vi "MAIN_TL_wait_cycle_end.vi"(6 "Gauge Refnum":refnum<vi>, 7 "# repetition":i32, 8 "error in":errorcluster, 9 "variant":variant, 10 "t0":dbl, 11 "# cycle":i32) -> (0 "error out":errorcluster, 1 "task":T1, 4 "# cycles":i32, 5 "To":dbl)   [LabVIEW 2015]
uses:
  CONTROLS/Q_main_element.ctl
  GLOBAL/Global_ABORT.vi
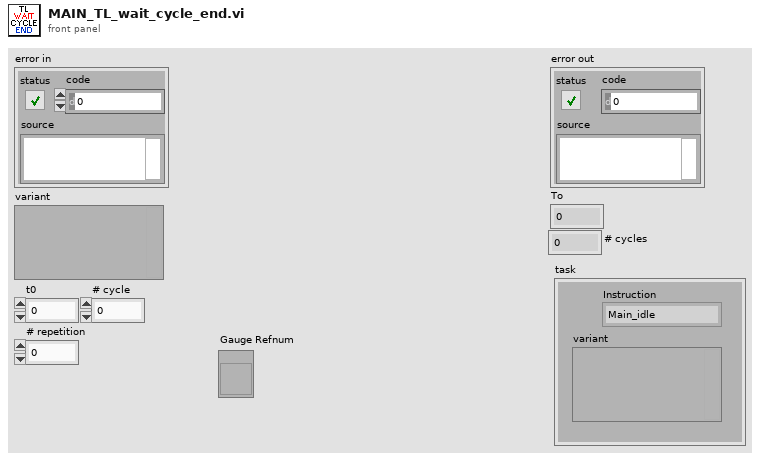
[diagram p1: front panel]
types:
  T1 = typedef "Q_main_element.ctl" = cluster{"variant":variant, "Instruction":enum16{"Main_idle", "Main_initialize", "Main_initialize_TDMS", "Main_initialize_Queue", "Main_error", "Main_DAQ_initialization_results", "Main_ASI_initialization_results", "Main_Piezo_initialization_results", "Main_Valve_initialization_results", "Main_Pump_initialization_results", "Main_CAMERA_initialization_results", "Main_DAQ_error", "Main_ASI_error", "Main_Piezo_error", "Main_CAMERA_error", "Main_Valve_error", "Main_Pump_error", "Main_start_acquiring", "Main_not_acquiring", "Main_acquiring", "Main_stop_acquiring", "Main_change_exposure", "Main_change_z_scan_parameters", "Main_define_ROI", "Main_define_mosaic", "Main_read_kinetic_time", "Main_cooler", "Main_read_temperature", "Main_save_XY", "Main_load_XY", "Main_discard_XY", "Main_move_to_XY", "Main_measure_QPD", "Main_autofocus_calibration", "Main_save_PID", "Main_change_H_valve_position", "Main_two_way_valve", "Main_save_movie", "Main_init_single_scan", "Main_single_scan", "Main_stop_single_scan", "Main_merFISH_illumination_parameters", "Main_merFISH_buffer_probe_list", "Main_merFISH_injections_procedure", "Main_merFISH_save_setpoint", "Main_merFISH_DAPI_parameters", "Main_merFISH_Brightfield_parameters", "Main_merFISH_save_embryo_ROI", "Main_merFISH_init", "Main_merFISH_resume", "Main_merFISH_start_autofocus", "Main_merFISH_open_close_valve_merFISH", "Main_merFISH_open_close_valve_photobleaching", "Main_merFISH_hybridization", "Main_merFISH_move_to_ROI", "Main_merFISH_wait_stabilization", "Main_merFISH_scan_laser", "Main_merFISH_scan_brightfield", "Main_merFISH_photobleaching_injection", "Main_merFISH_photobleaching", "Main_merFISH_save", "Main_merFISH_send_email", "Main_merFISH_close", "Main_TL_define_parameters", "Main_TL_reset_parameters", "Main_TL_init", "Main_TL_start_autofocus", "Main_TL_move_to_ROI", "Main_TL_wait_for_stabilization", "Main_TL_scan", "Main_TL_wait_cycle_end", "Main_TL_close", "Main_STOP"}}
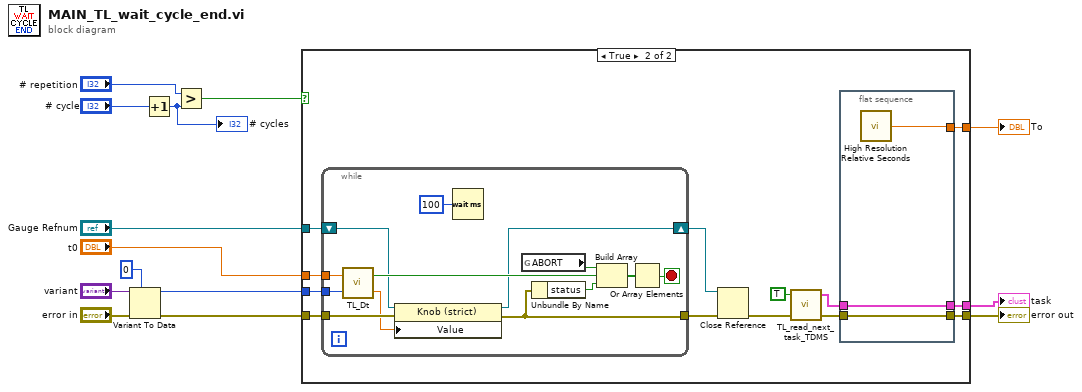
[diagram p0: block diagram]
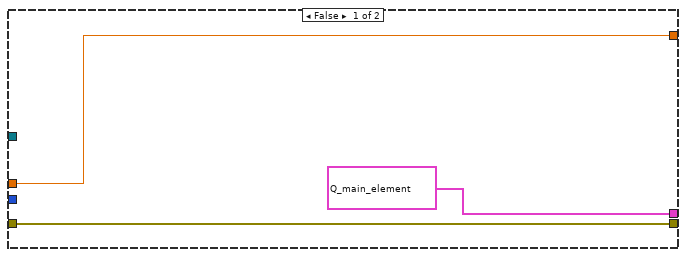
[diagram p2: hidden frame]
diagram:
  n1 = Variant To Data(error in="error in", type=0 ("Dt (s)"), Variant="variant") -> (data=w13:i32, error out=w14:errorcluster)
  n2 = Increment(x="# cycle") -> (x+1=w2:i32)
  "# cycles" <- w2
  n3 = Greater?(x="# repetition", y=w2) -> (0:w12:bool)
  n4 = case shown="True" w12 {
    tunnel: w13 -> [_ w30]
    tunnel: "t0" -> [w15 w29]
    tunnel: w14 -> [w17 w28]
    tunnel: [w15 w25] -> w6
    tunnel: [T1 {"variant"=variant, "Instruction"=enum."Main_TL_close"} ("task") w24] -> w7
    tunnel: [w17 w23] -> w8
    tunnel: "Gauge Refnum" -> [_ w21]
    frame False {
    }
    frame True {
      n5 = while {
        tunnel: w28 -> [w38]
        tunnel: w30 -> [w46]
        tunnel: w29 -> [w39]
        tunnel: [w34] -> w20
        shift-right: [w35] -> w19
        shift-left: w21 -> [w37]
        stop <- w41 stop-if-true
        n6 = call "TL_Dt.vi"("Dt (s)"=w46, "t0"=w39) -> ("Gauge"=w36:dbl, "STOP"=w44:bool)
        n7 = property class="Knob (strict)"(reference=w37, error in=w38, "Value"=w36) -> (reference out=w35:refnum<vi>, error out=w34:errorcluster)
        n8 = Wait (ms)(milliseconds to wait=u32 100) -> ()  [unwired: 1 out]
        n9 = global read "Global_ABORT.vi" "ABORT"() -> (w43:bool)
        n10 = Unbundle By Name(w34) -> ("status"=w40:bool)
        n11 = Build Array(w43, w44, w40) -> (w42:bool[])
        n12 = Or Array Elements(Boolean array=w42) -> (logical OR=w41:bool)
      }
      n13 = Close Reference(reference=w19, error in (no error)=w20) -> (error out=w18:errorcluster)
      n14 = call "TL_read_next_task_TDMS.vi"("error in"=w18, "Reset"=TRUE) -> ("error out"=w26:errorcluster, "task"=w27:T1)  [unwired: 2 in]
      n15 = flat-sequence {
        tunnel: w26 -> [w33]
        tunnel: [w33] -> w23
        tunnel: w27 -> [w32]
        tunnel: [w32] -> w24
        tunnel: [w31] -> w25
        frame #0 {
          n16 = call <vilib>:"High Resolution Relative Seconds.vi"() -> ("relative seconds"=w31:dbl)
        }
      }
    }
  }
  "error out" <- w8
  "task" <- w7
  "To" <- w6
